vi "文件路径（通用）.vi"() -> ()   [LabVIEW 2018]
panel:
  out "添加的路径":path
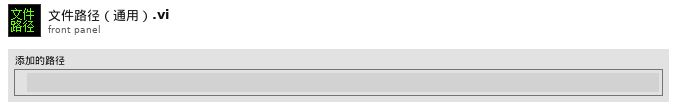
[diagram p1: front panel]
types:
  T1 = enum32{"invalid app kind", "Development System", "Run Time System", "Student Edition", "Embedded LabVIEW", "Evaluation", "Custom"}
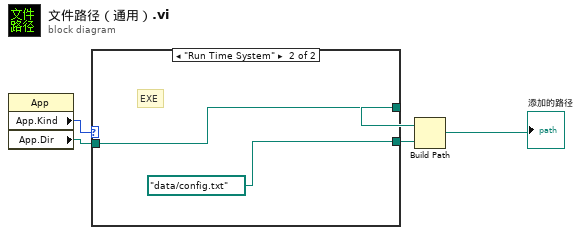
[diagram p0: block diagram]
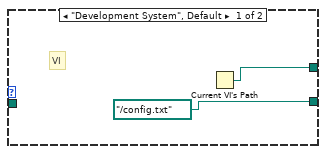
[diagram p2: hidden frame]
diagram:
  n1 = property class="App"() -> ("App.Kind"=w3:T1, "App.Dir"=w2:path)  [unwired: 2 in, 2 out]
  n2 = case shown="\"Run Time System\"" w3 {
    tunnel: [w6 w9] -> w4
    tunnel: w2 -> [_ w9]
    tunnel: [path "../config.txt" ("App.Dir") path "data/config.txt" ("App.Dir")] -> w1
    frame "Development System", Default {
      # "VI"
      n3 = Current VI's Path() -> (path=w6:path)
    }
    frame "Run Time System" {
      # "EXE"
    }
  }
  n4 = Build Path(base path=w4, name or relative path=w1) -> (appended path=→"添加的路径":path)
